vi "File updated.vi"(8 "error in (no error)":errorcluster, 10 "File Path Control":path, 11 "Plot in":refnum<class "Plot.lvclass">) -> (0 "error out":errorcluster, 3 "Plot out":refnum<class "Plot.lvclass">)   [LabVIEW 2016, in "Plot.lvclass"]
uses:
  Plot.lvclass
  Plot.lvclass/Plot.ctl
  Read Files.vi
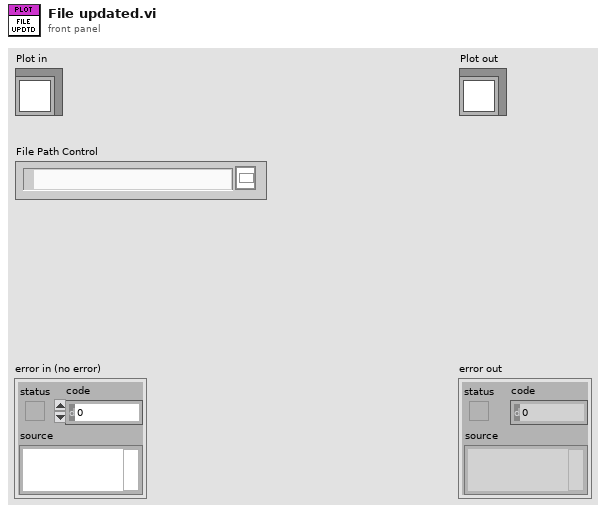
[diagram p1: front panel]
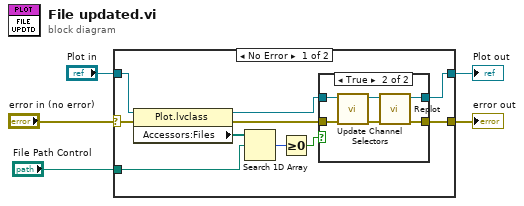
[diagram p0: block diagram]
diagram:
  n1 = case shown="No Error" "error in (no error)" {
    selector: "error in (no error)" -> [w8 w25]
    tunnel: [w7 w25] -> w4
    tunnel: [w10 w24] -> w2
    tunnel: "Plot in" -> [w15 w24]
    tunnel: "File Path Control" -> [w12 _]
    frame No Error {
      n2 = property class="Plot.lvclass"(reference=w15, error in=w8) -> (reference out=w14:refnum<class "Plot.lvclass">, error out=w9:errorcluster, "Accessors:Files"=w13:path[])
      n3 = Search 1D Array(1D array=w13, element=w12) -> (index of element=w11:i32)  [unwired: 1 in]
      n4 = Greater Or Equal To 0?(x=w11) -> (x >= 0?=w6:bool)
      n5 = case shown="True" w6 {
        tunnel: w14 -> [w17 w23]
        tunnel: [w17 w22] -> w10
        tunnel: w9 -> [w16 w19]
        tunnel: [w16 w21] -> w7
        frame False {
        }
        frame True {
          n6 = call-dynamic "Update Channel Selectors.vi"("error in (no error)"=w19, "Plot in"=w23) -> ("error out"=w18:errorcluster, "Plot out"=w20:refnum<class "Plot.lvclass">)  [unwired: 8 in]
          n7 = call-dynamic "Replot.vi"("error in (no error)"=w18, "Plot in"=w20) -> ("error out"=w21:errorcluster, "Plot out"=w22:refnum<class "Plot.lvclass">)  [unwired: 8 in]
        }
      }
    }
    frame Error {
    }
  }
  "error out" <- w4
  "Plot out" <- w2
